vi "rATE SCAN FIND OFFSET CREATE ARRAY.vi"(0 "THx":u16, 1 "HLTHx":dbl, 2 "Scaler 2":u16, 3 "LVDS HLTH":bool, 4 "TH":u16[](array[numeric]), 5 "VTH":dbl[](array[numeric]), 6 "Scaler":u16[](array[numeric]), 7 "LVDS":bool[](array[boolean]), 8 "In Range":bool) -> (24 "THo":u16[](array[numeric]), 25 "VTHo":dbl[](array[numeric]), 26 "Scalero":u16[](array[numeric]), 27 "LVDSo":bool[](array[boolean]))   [LabVIEW 2009]
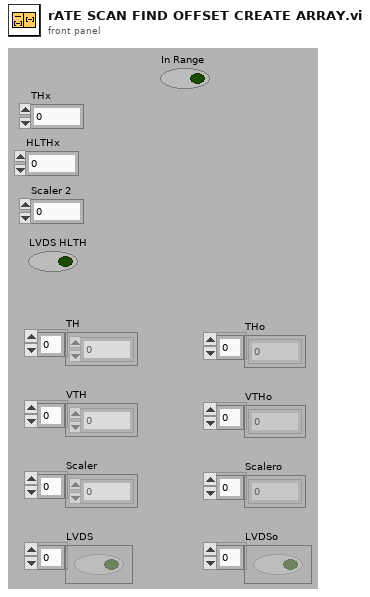
[diagram p1: front panel]
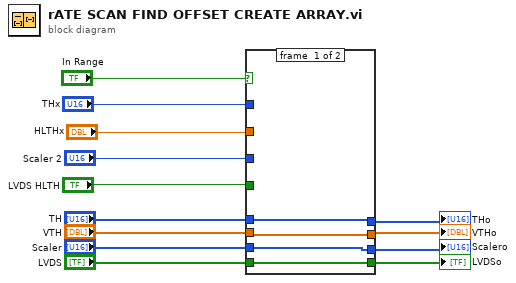
[diagram p0: block diagram]
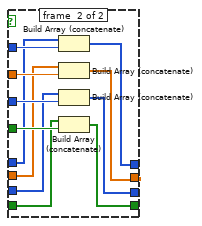
[diagram p2: hidden frame]
diagram:
  n1 = case shown="True" "In Range" {
    tunnel: "LVDS HLTH" -> [_ w29]
    tunnel: "Scaler 2" -> [_ w28]
    tunnel: "HLTHx" -> [_ w27]
    tunnel: "THx" -> [_ w26]
    tunnel: [w17 w25] -> w10
    tunnel: [w16 w24] -> w11
    tunnel: [w15 w23] -> w12
    tunnel: [w14 w22] -> w13
    tunnel: "TH" -> [w17 w21]
    tunnel: "VTH" -> [w16 w20]
    tunnel: "Scaler" -> [w15 w19]
    tunnel: "LVDS" -> [w14 w18]
    frame #0 {
    }
    frame #1 {
      n2 = Build Array (concatenate)(w21, w26) -> (w25:u16[])
      n3 = Build Array (concatenate)(w20, w27) -> (w24:dbl[])
      n4 = Build Array (concatenate)(w19, w28) -> (w23:u16[])
      n5 = Build Array (concatenate)(w18, w29) -> (w22:bool[])
    }
  }
  "LVDSo" <- w13
  "Scalero" <- w12
  "VTHo" <- w11
  "THo" <- w10
